vi "example_2_6_c.vi"() -> ()   [LabVIEW 2018]
panel:
  in  "Ring":u16(ring) items=["my option", "option 2", "option 3"]
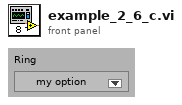
[diagram p1: front panel]
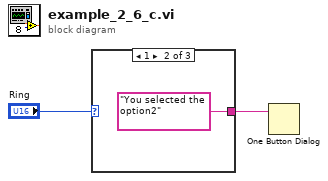
[diagram p0: block diagram]
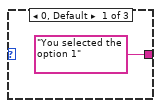
[diagram p2: hidden frame]
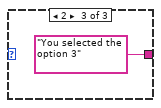
[diagram p3: hidden frame]
diagram:
  n1 = case shown="1" "Ring" {
    tunnel: ["You selected the option 1" "You selected the option2" "You selected the option 3"] -> w1
    frame 0, Default {
    }
    frame 1 {
    }
    frame 2 {
    }
  }
  n2 = One Button Dialog(message=w1) -> ()  [unwired: 1 in, 1 out]
